vi "Init.vi"(4 "Message Cfg":T1={"EnTermChar"=TRUE, "termChar"=10, "suppEnEnRd"=FALSE, "sendEndEn"=FALSE} {"termChar" format="%.0x"}, 6 "timeout":u32=1000, 7 "Name":string, 8 "error in":errorcluster, 9 "serialCfg":T2={"baud rate (9600)"=9600, "data bits (8)"=8, "stop bits (10: 1 bit)"=10, "parity (0:none)"=enum."None", "flow control (0:none)"=0, "endModeforReads"=0, "endModeforWrites"=0} {"endModeforWrites" items=["None", "Last Bit", "TermChar", "Break"]; "endModeforReads" items=["None", "Last Bit", "TermChar"]; "flow control (0:none)" items=["None", "XON/XOFF", "RTS/CTS", "XON/XOFF & RTS/CTS", "DTR/DSR", "XON/XOFF & DTR/DSR"]; "stop bits (10: 1 bit)" items=["1.0"=10, "1.5"=15, "2.0"=20]; "data bits (8)" min=5 max=8 step=1}, 10 "Port":refnum<visa-resource-name>, 11 "Serial IO in":refnum<class "Serial IO.lvclass">) -> (0 "error out":errorcluster, 3 "Serial IO out":refnum<class "Serial IO.lvclass">)   [LabVIEW 2015, in "Serial IO.lvclass"]
doc: "Initialize communication with a serial port. Open the port and obtain a reference to a semaphore that will be used to prevent communication clashes. If the device is recorded as \"present\" at initialization, then the port will be closed and initialization will then proceed as intended."
uses:
  Serial IO.lvclass
  Serial IO.lvclass/Serial IO.ctl
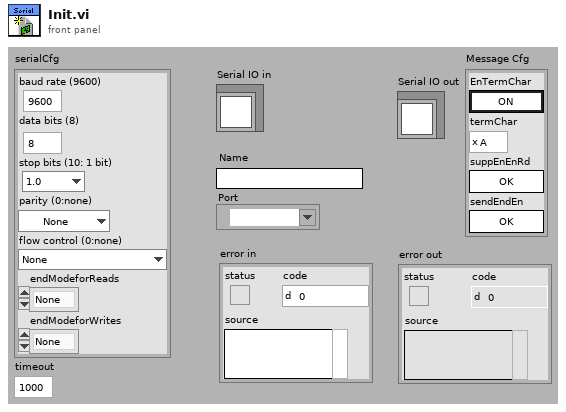
[diagram p1: front panel]
types:
  T1 = cluster{"EnTermChar":bool, "termChar":u8, "suppEnEnRd":bool, "sendEndEn":bool}
  T2 = cluster{"baud rate (9600)":u32, "data bits (8)":u16, "stop bits (10: 1 bit)":u16, "parity (0:none)":enum16{"None", "Odd", "Even", "Mark", "Space"}, "flow control (0:none)":u16, "endModeforReads":u16, "endModeforWrites":u16}
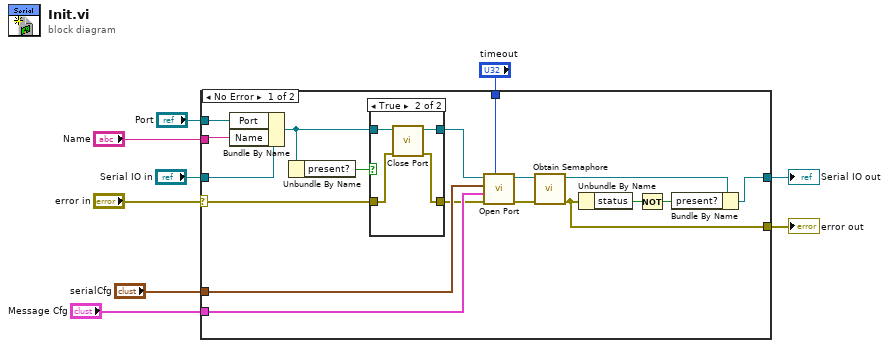
[diagram p0: block diagram]
diagram:
  n1 = case shown="No Error" "error in" {
    selector: "error in" -> [w11 w34]
    tunnel: "Serial IO in" -> [w27 w35]
    tunnel: [w21 w35] -> w7
    tunnel: [w20 w34] -> w6
    tunnel: "Port" -> [w19 _]
    tunnel: "Name" -> [w25 _]
    tunnel: "serialCfg" -> [w17 _]
    tunnel: "Message Cfg" -> [w15 _]
    tunnel: "timeout" -> [w16 _]
    frame No Error {
      n2 = Bundle By Name(cluster=w27, "Port"=w19, "Name"=w25) -> (w13:refnum<class "Serial IO.lvclass">)
      n3 = Unbundle By Name(w13) -> ("present?"=w14:bool)
      n4 = case shown="True" w14 {
        tunnel: w13 -> [w29 w33]
        tunnel: [w29 w32] -> w12
        tunnel: w11 -> [w28 w31]
        tunnel: [w28 w30] -> w10
        frame False {
        }
        frame True {
          n5 = call-dynamic "Close Port.vi"("error in (no error)"=w31, "Serial IO in"=w33) -> ("error out"=w30:errorcluster, "Serial IO out"=w32:refnum<class "Serial IO.lvclass">)  [unwired: 8 in]
        }
      }
      n6 = call "Open Port.vi"("timeout"=w16, "error in"=w10, "Message Cfg"=w15, "serialCfg"=w17, "Serial IO in"=w12) -> ("error out"=w18:errorcluster, "Serial IO out"=w26:refnum<class "Serial IO.lvclass">)  [unwired: 5 in]
      n7 = call "Obtain Semaphore.vi"("error in"=w18, "Serial IO in"=w26) -> ("error out"=w20:errorcluster, "Serial IO out"=w23:refnum<class "Serial IO.lvclass">)  [unwired: 8 in]
      n8 = Unbundle By Name(w20) -> ("status"=w24:bool)
      n9 = Not(x=w24) -> (.not. x?=w22:bool)
      n10 = Bundle By Name(cluster=w23, "present?"=w22) -> (w21:refnum<class "Serial IO.lvclass">)
    }
    frame Error {
    }
  }
  "error out" <- w6
  "Serial IO out" <- w7
